vi "DestroyRequestEvents.vi"(8 "error in (no error)":errorcluster) -> (0 "error out":errorcluster)   [LabVIEW 2014, in "FGenModule.lvlib"]
uses:
  FGenModule.lvlib
  clRequestEvents.ctl
  clEventType.ctl
panel:
  out "clRequestEvents":T1
  # "If you want to add other Request Events, open this typedef, copy an existing event and rename it to your Request name.\n\nNext create a typedef for the  data and put it into PublicAPI/Arguments/Requests\n\nNext, add an event handler loop event case in Main.vi to handle the new request event\n\nMost likely, each request will also require the creation of a new Queued Message Handler loop case in Main.VI"
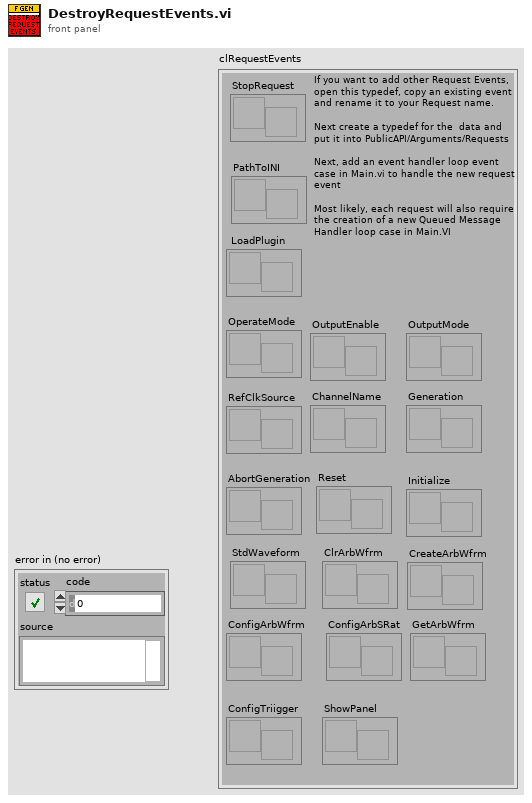
[diagram p1: front panel]
types:
  T1 = typedef "FGenModule.lvlib/clRequestEvents.ctl" = cluster{"StopRequest":refnum<user-event>, "PathToINI":refnum<user-event>, " LoadPlugin":refnum<user-event>, "OperateMode":refnum<user-event>, "OutputEnable":refnum<user-event>, "OutputMode":refnum<user-event>, "RefClkSource":refnum<user-event>, "ChannelName":refnum<user-event>, "Generation":refnum<user-event>, "AbortGeneration":refnum<user-event>, "Reset":refnum<user-event>, "Initialize":refnum<user-event>, "StdWaveform":refnum<user-event>, "ClrArbWfrm":refnum<user-event>, "CreateArbWfrm":refnum<user-event>, "ConfigArbWfrm":refnum<user-event>, "ConfigArbSRat":refnum<user-event>, "GetArbWfrm":refnum<user-event>, "ConfigTriigger":refnum<user-event>, "ShowPanel":refnum<user-event>}
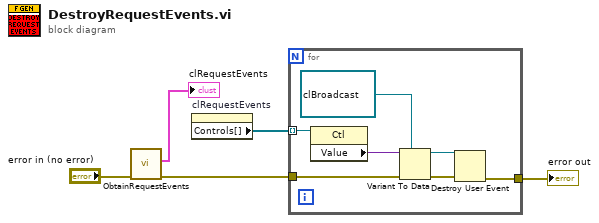
[diagram p0: block diagram]
diagram:
  n1 = call "ObtainRequestEvents.vi"("error in (no error)"="error in (no error)") -> ("error out"=w2:errorcluster, "clRequestEvents"=→"clRequestEvents":T1)  [unwired: 9 in]
  n2 = property on="clRequestEvents" class="Clust (strict)"() -> ("Controls[]"=w4:refnum<vi>[])  [unwired: 2 in, 2 out]
  n3 = for {
    tunnel: w4 -> [w12] mode=indexing
    tunnel: w2 -> [w9]
    tunnel: [w8] -> w5
    n4 = property class="Ctl"(reference=w12) -> ("Value"=w11:variant)  [unwired: 1 in, 2 out]
    n5 = Variant To Data(error in=w9, type=refnum<user-event> refnum ("StopRequest"), Variant=w11) -> (data=w7:refnum<user-event>, error out=w10:errorcluster)
    n6 = Destroy User Event(user event=w7, error in=w10) -> (error out=w8:errorcluster)
  }
  "error out" <- w5
